vi "getPosMouse.vi"() -> (0 "y":i32, 1 "x":i32)   [LabVIEW 2020]
uses:
  <vilib>/Utility/inputDevices.llb/mouseAcquire.vi
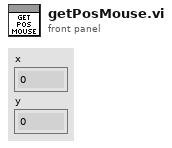
[diagram p1: front panel]
types:
  T1 = cluster{"Horizontal":i32, "Vertical":i32, "Scrolling":i32}
  T2 = typedef "LVPointTypeDef.ctl" = cluster{"Horizontal":i16, "Vertical":i16}
  T3 = typedef "LVRectTypeDef.ctl" = cluster{"Left":i16, "Top":i16, "Right":i16, "Bottom":i16}
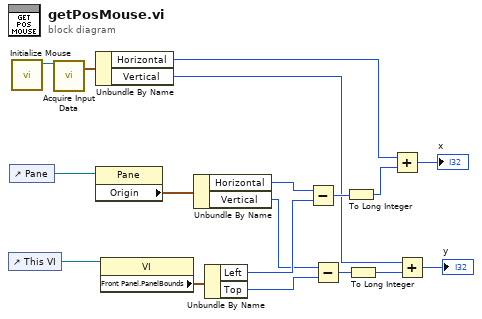
[diagram p0: block diagram]
diagram:
  n1 = control-ref of="This VI"() -> (w16:refnum<vi>)
  n2 = control-ref of="Pane"() -> (w18:refnum<vi>)
  n3 = call <vilib>:"Initialize Mouse.vi"() -> ("device ID"=w8:refnum<k1>)  [unwired: 10 in, 1 out]
  n4 = call-poly <vilib>:"Acquire Input Data.vi"("device ID"=w8) -> ("axis info"=w7:T1)  [unwired: 15 in, 3 out]
  n5 = Unbundle By Name(w7) -> ("Horizontal"=w5:i32, "Vertical"=w3:i32)
  n6 = property class="Pane"(reference=w18) -> ("Origin"=w17:T2)  [unwired: 1 in, 2 out]
  n7 = property class="VI"(reference=w16) -> ("Front Panel.PanelBounds"=w15:T3)  [unwired: 1 in, 2 out]
  n8 = Unbundle By Name(w17) -> ("Horizontal"=w14:i16, "Vertical"=w12:i16)
  n9 = Unbundle By Name(w15) -> ("Left"=w13:i16, "Top"=w11:i16)
  n10 = Subtract(x=w14, y=w13) -> (x-y=w10:i16)
  n11 = Subtract(x=w12, y=w11) -> (x-y=w9:i16)
  n12 = To Long Integer(number=w10) -> (32bit integer=w6:i32)
  n13 = To Long Integer(number=w9) -> (32bit integer=w4:i32)
  n14 = Add(x=w5, y=w6) -> (x+y=→"x":i32)
  n15 = Add(x=w3, y=w4) -> (x+y=→"y":i32)
